vi "TempConfigurationSubVI.vi"(8 "error in":errorcluster, 10 "Sim?":bool, 11 "physical channels":tag) -> (0 "error out":errorcluster, 3 "temperature task out":refnum<k21> caption="task out")   [LabVIEW 2015]
uses:
  <vilib>/DAQmx/create/channels.llb/DAQmx Create Channel (AI-Temperature-Thermocouple).vi
  <vilib>/DAQmx/configure/timing.llb/DAQmx Timing (Sample Clock).vi
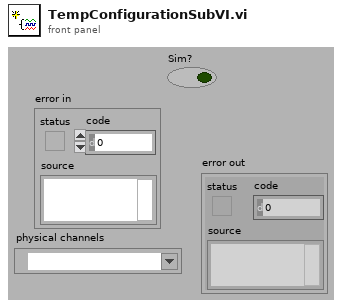
[diagram p1: front panel]
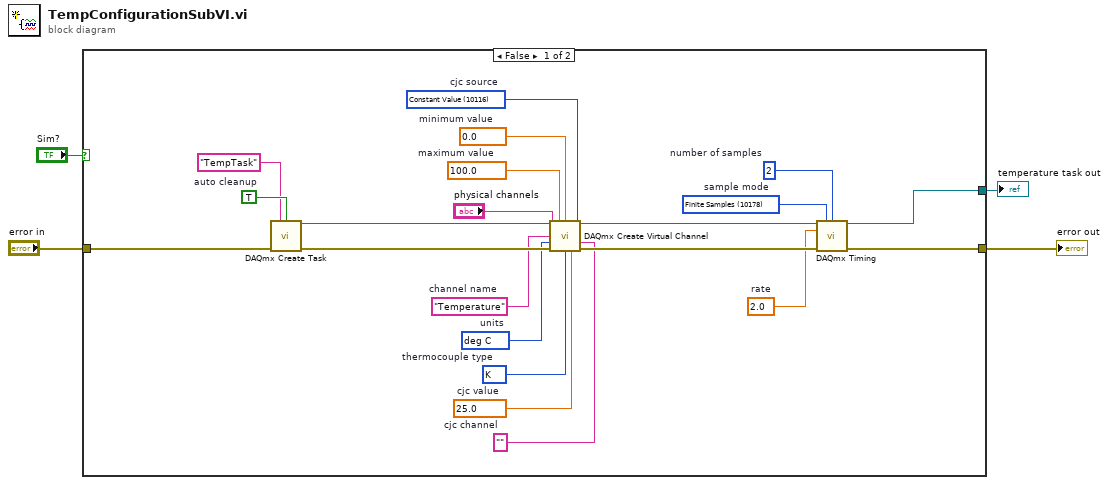
[diagram p0: block diagram]
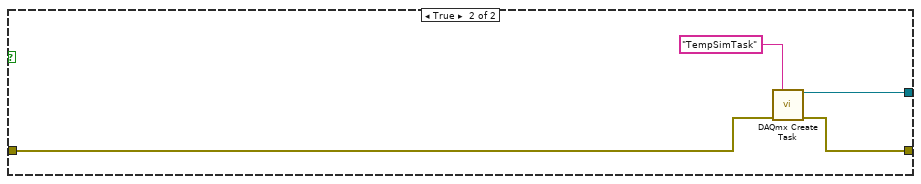
[diagram p2: hidden frame]
diagram:
  n1 = case shown="False" "Sim?" {
    tunnel: "error in" -> [w25 w26]
    tunnel: [w12 w28] -> w3
    tunnel: [w5 w27] -> w1
    frame False {
      w8 = 10178 items=["Finite Samples"=10178, "Continuous Samples"=10123, "Hardware Timed Single Point"=12522]  # sample mode
      w9 = 2  # number of samples
      w10 = 2.0  # rate
      w13 = 10116 items=["Built-In"=10200, "Constant Value"=10116, "Channel"=10113]  # cjc source
      w15 = ""  # cjc channel
      w16 = 25.0  # cjc value
      w17 = 10073 items=["J"=10072, "K"=10073, "N"=10077, "R"=10082, "S"=10085, "T"=10086, "B"=10047, "E"=10055]  # thermocouple type
      w18 = 10143 items=["deg C"=10143, "deg F"=10144, "Kelvins"=10325, "deg R"=10145, "From Custom Scale"=10065]  # units
      w14 = "Temperature"  # channel name
      w20 = 0.0  # minimum value
      w21 = 100.0  # maximum value
      w23 = TRUE  # auto cleanup
      n2 = call <vilib>:"DAQmx Create Task.vi"("new task name"="TempTask", "auto cleanup"=w23, "error in"=w25) -> ("task out"=w22:refnum<k21>, "error out"=w24:errorcluster)  [unwired: 11 in]
      n3 = call-poly <vilib>:"DAQmx Create Virtual Channel.vi"("task in"=w22, "maximum value"=w21, "minimum value"=w20, "physical channels"="physical channels", "cjc source"=w13, "name to assign"=w14, "units"=w18, "cjc channel"=w15, "error in"=w24, "thermocouple type"=w17, "cjc value"=w16) -> ("task out"=w11:refnum<k21>, "error out"=w19:errorcluster)  [unwired: 3 in]
      n4 = call-poly <vilib>:"DAQmx Timing.vi"("task/channels in"=w11, "sample mode"=w8, "samples per channel"=w9, "rate"=w10, "error in"=w19) -> ("task out"=w12:refnum<k21>, "error out"=w5:errorcluster)  [unwired: 9 in]
    }
    frame True {
      n5 = call <vilib>:"DAQmx Create Task.vi"("new task name"="TempSimTask", "error in"=w26) -> ("task out"=w28:refnum<k21>, "error out"=w27:errorcluster)  [unwired: 12 in]
    }
  }
  "temperature task out" <- w3
  "error out" <- w1
